vi "Initialize.vi"(6 "Start Direction":T1=enum."E", 8 "error in (no error)":errorcluster, 9 "Kamikaze DVR":T2, 10 "SquareStatus DVR":T3, 11 "Coward in":refnum<class "Coward.lvclass">) -> (0 "error out":errorcluster, 3 "Coward out":refnum<class "Coward.lvclass">)   [LabVIEW 2015, in "Coward.lvclass"]
uses:
  Coward.lvclass
  Formics/SquareStatus DVR.ctl
  Formics/Kamikaze DVR.ctl
  Type Defs/Direction Enum.ctl
  Coward.lvclass/Coward.ctl
  Formics/Formics.lvclass
  Type Defs/SB Type Defs.lvlib
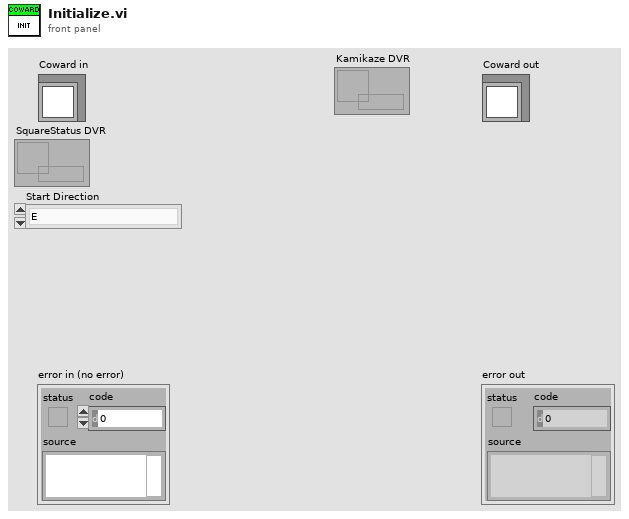
[diagram p1: front panel]
types:
  T1 = typedef "SB Type Defs.lvlib/Direction Enum.ctl" = enum16{"NW", "N", "NE", "E", "SE", "S", "SW", "W"}
  T2 = typedef "Formics.lvclass/Kamikaze DVR.ctl" = refnum<data-value>
  T3 = typedef "Formics.lvclass/SquareStatus DVR.ctl" = refnum<data-value>
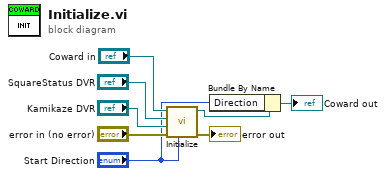
[diagram p0: block diagram]
diagram:
  n1 = call-parent "Initialize.vi"("Start Direction"="Start Direction", "error in (no error)"="error in (no error)", "Kamikaze DVR"="Kamikaze DVR", "SquareStatus DVR"="SquareStatus DVR", "Mother in"="Coward in") -> ("error out"=→"error out":errorcluster, "Mother out"=w7:refnum<class "Coward.lvclass">)  [unwired: 5 in]
  n2 = Bundle By Name(cluster=w7, "Direction"="Start Direction") -> (→"Coward out":refnum<class "Coward.lvclass">)
